vi "Pulse Attribute, Calculate Chart Zoom.vi"(8 "error in":errorcluster, 11 "waveform":waveform(dbl)={"t0"=timestamp(3473168073.631 s since 1904-01-01), "dt"=1e-08, "Y"=[], "attributes"=variant("Average Size"=variant(dbl 15.0), "Frequency (Hz)"=variant(dbl 1997.9906429610444), "NSamp"=variant(dbl 400000.0), "Recvy Amp (mA)"=variant(dbl 5.267865023873527), "Recvy Amp (mV)"=variant(dbl 2633.932511936763), "Recvy Frequency (Hz)"=variant(dbl 1998.1395072914302), "Recvy Pulse Width (us)"=variant(dbl 12.427603778839112), "Recvy Trigger (s)"=variant(dbl 0.00043972), "Resistance (ohms)"=variant(dbl 500.0), "Samp Freq (MHz)"=variant(dbl 100.0), "Stim Amp (mA)"=variant(dbl -4.607747165232184), "Stim Amp (mV)"=variant(dbl -2303.873582616092), "Stim Frequency (Hz)"=variant(dbl 1997.8417786306586), "Stim Pulse Width (us)"=variant(dbl 12.076313257217407), "Stim Trigger (s)"=variant(dbl 0.00041185), "dt (us)"=variant(dbl 0.01))}) -> (0 "error out":errorcluster, 1 "X Scale:Max":dbl=nan format="%.3p", 2 "X Scale:Min":dbl=nan format="%.3p", 3 "waveform dup":waveform(dbl)={"t0"=timestamp(0 s since 1904-01-01), "dt"=nan, "Y"=[]}, 4 "Stim Amp (V)":dbl=nan format="%.1f", 5 "Stim Trigger (s)":dbl=nan format="%.3p", 6 "Recvy Amp (V)":dbl=nan format="%.1f", 7 "Recvy Trigger (s)":dbl=nan format="%.3p")   [LabVIEW 2010]
panel:
  # "Indicator order is optimized for wiring to the Set Cursor.vi"
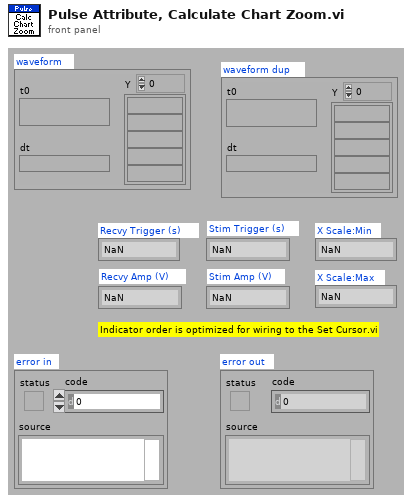
[diagram p1: front panel]
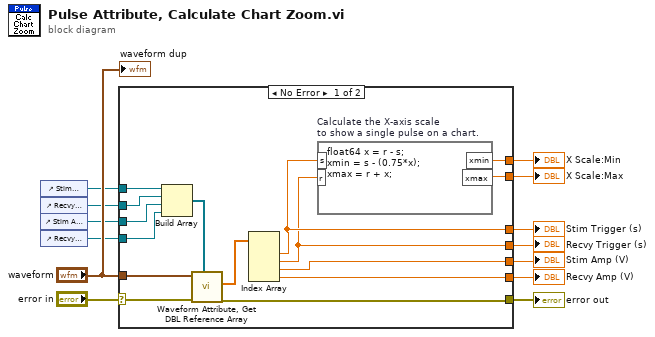
[diagram p0: block diagram]
diagram:
  n1 = control-ref of="Stim Trigger (s)"() -> (w8:refnum<vi>)
  n2 = control-ref of="Recvy Trigger (s)"() -> (w7:refnum<vi>)
  n3 = control-ref of="Stim Amp (V)"() -> (w6:refnum<vi>)
  n4 = control-ref of="Recvy Amp (V)"() -> (w5:refnum<vi>)
  n5 = case shown="No Error" "error in" {
    selector: "error in" -> [w26 w29]
    tunnel: "waveform" -> [w23 _]
    tunnel: [w28 _] -> w12
    tunnel: [w27 _] -> w11
    tunnel: [w19 w29] -> w10
    tunnel: w8 -> [w25 _]
    tunnel: w7 -> [w24 _]
    tunnel: [w21 _] -> w3
    tunnel: [w20 _] -> w4
    tunnel: w6 -> [w18 _]
    tunnel: w5 -> [w17 _]
    tunnel: [w16 _] -> w1
    tunnel: [w15 _] -> w2
    frame No Error {
      n6 = Build Array(w25, w24, w18, w17) -> (w14:refnum<vi>[])
      n7 = call "Waveform Attribute, Get DBL Reference Array.vi"("refnum array"=w14, "error in"=w26, "waveform"=w23) -> ("error out"=w19:errorcluster, "values"=w22:dbl[])  [unwired: 2 in, 3 out]
      n8 = Index Array(array=w22) -> (element #1=w16:dbl, element #2=w15:dbl, element #3=w21:dbl, element #4=w20:dbl)  [unwired: 4 in]
      n9 = formula code="float64 x = r - s;\nxmin = s - (0.75*x);\nxmax = r + x;" "Calculate the X-axis scale\nto show a single pulse on a chart."("s"=w16, "r"=w15) -> ("xmin"=w27:dbl, "xmax"=w28:dbl)
    }
    frame Error {
    }
  }
  "error out" <- w10
  "X Scale:Min" <- w11
  "X Scale:Max" <- w12
  "Stim Trigger (s)" <- w1
  "Recvy Trigger (s)" <- w2
  "Recvy Amp (V)" <- w4
  "Stim Amp (V)" <- w3
  "waveform dup" <- "waveform"
